vi "Update Camera Modes.vi"(8 "error in (no error)":errorcluster, 10 "StringsAndValues":cluster{"String":string, "Value":i32}[](array[cluster]), 11 "Main Window in":refnum<class "Main Window.lvclass">) -> (0 "error out":errorcluster, 3 "Main Window out":refnum<class "Main Window.lvclass">)   [LabVIEW 2023, in "Main Window.lvlib" / "Main Window.lvclass"]
uses:
  Main Window.lvclass
  Main Window.lvclass/Main Window.ctl
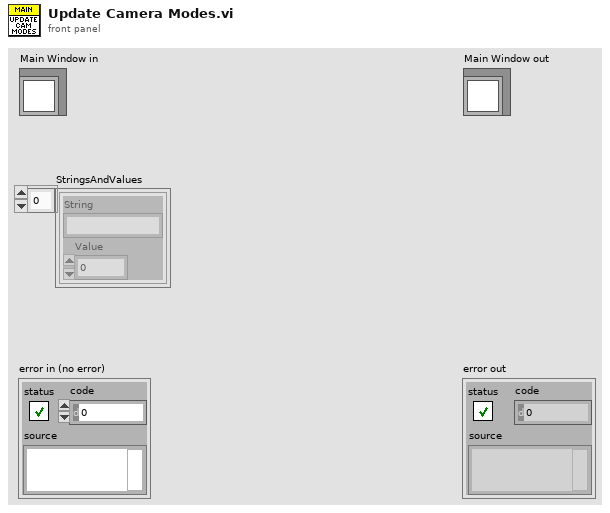
[diagram p1: front panel]
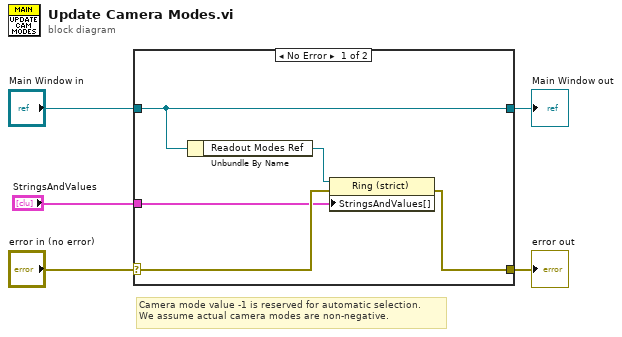
[diagram p0: block diagram]
diagram:
  # "Camera mode value -1 is reserved for automatic selection.\nWe assume actual camera modes are non-negative."
  n1 = case shown="No Error" "error in (no error)" {
    selector: "error in (no error)" -> [w8 w12]
    tunnel: [w7 w12] -> w4
    tunnel: [w10 w11] -> w2
    tunnel: "Main Window in" -> [w10 w11]
    tunnel: "StringsAndValues" -> [w6 _]
    frame No Error {
      n2 = Unbundle By Name(w10) -> ("Readout Modes Ref"=w9:refnum<vi>)
      n3 = property class="Ring (strict)"(reference=w9, error in=w8, "StringsAndValues[]"=w6) -> (error out=w7:errorcluster)  [unwired: 1 out]
    }
    frame Error {
    }
  }
  "error out" <- w4
  "Main Window out" <- w2
